vi "MTMount_putSample_Elevation.vi"(8 "error in (no error)":errorcluster, 11 "Elevation_Ctl":T1) -> (0 "error out":errorcluster, 2 "function return":i32, 3 "Elevation_Ctl out":T1)   [LabVIEW 2018, in "SALLV_MTMount.lvlib"]
doc: "int MTMount_shm_putSample_ElevationLV(MTMount_ElevationLV *Elevation_Ctl );"
uses:
  SALLV_MTMount.lvlib
  DataTypes/Elevation.ctl
  SALLV_MTMount.so
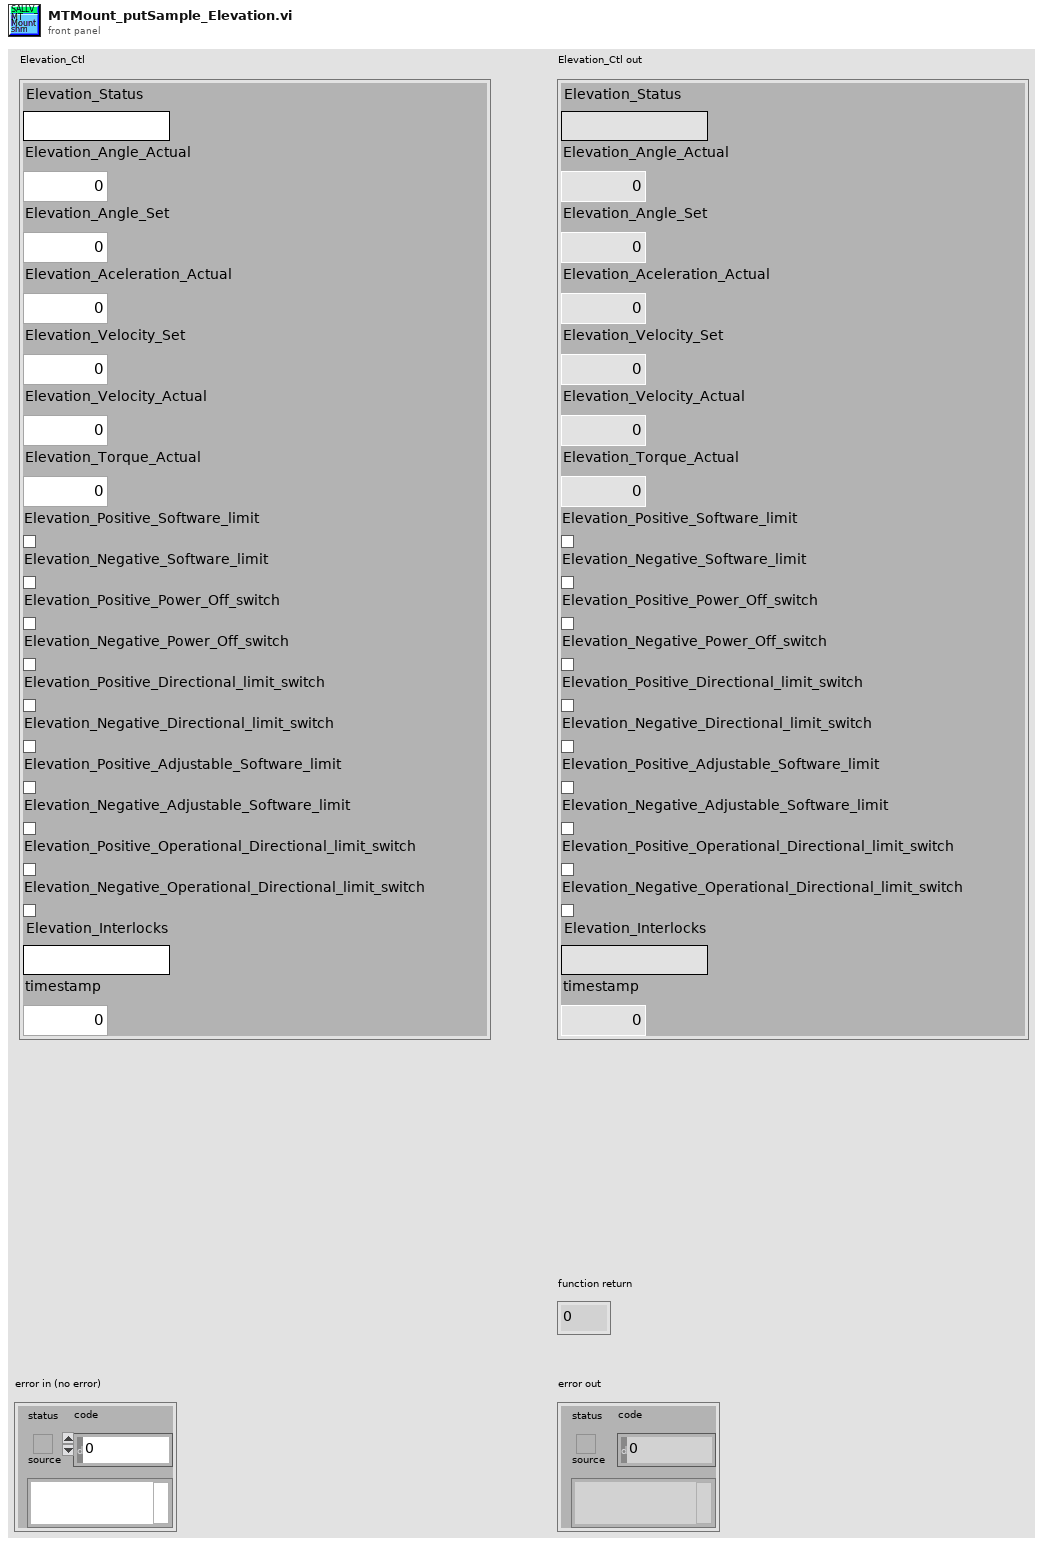
[diagram p1: front panel]
types:
  T1 = typedef "SALLV_MTMount.lvlib/Elevation.ctl" = cluster{"Elevation_Status":string, "Elevation_Angle_Actual":dbl, "Elevation_Angle_Set":dbl, "Elevation_Aceleration_Actual":dbl, "Elevation_Velocity_Set":dbl, "Elevation_Velocity_Actual":dbl, "Elevation_Torque_Actual":dbl, "Elevation_Positive_Software_limit":bool, "Elevation_Negative_Software_limit":bool, "Elevation_Positive_Power_Off_switch":bool, "Elevation_Negative_Power_Off_switch":bool, "Elevation_Positive_Directional_limit_switch":bool, "Elevation_Negative_Directional_limit_switch":bool, "Elevation_Positive_Adjustable_Software_limit":bool, "Elevation_Negative_Adjustable_Software_limit":bool, "Elevation_Positive_Operational_Directional_limit_switch":bool, "Elevation_Negative_Operational_Directional_limit_switch":bool, "Elevation_Interlocks":string, "timestamp":dbl}
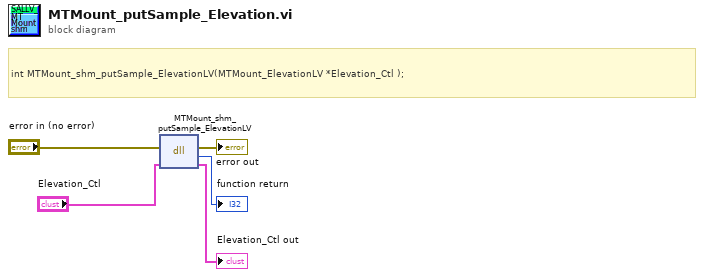
[diagram p0: block diagram]
diagram:
  # "int MTMount_shm_putSample_ElevationLV(MTMount_ElevationLV *Elevation_Ctl );"
  n1 = dll-call lib="home/ttsai/Document/salApiMTMount/SALLV_MTMount/SALLV_MTMount.*" fn="MTMount_shm_putSample_ElevationLV"(error in="error in (no error)", "Elevation_Ctl"="Elevation_Ctl") -> (error out=→"error out":errorcluster, →"function return":i32, "Elevation_Ctl"=→"Elevation_Ctl out":T1)  [unwired: 2 in, 1 out]
